vi "recenter.vi"() -> ()   [LabVIEW 2011]
doc: "This VI is an example of how to use the Host VI to open the I2C bus, write, read, and close I2C bus. This VI should work for any I2C EEPROM or RAM IC. Note that many of these devices have a limit on how many bytes can be writen to the device at a time.\n\nWritten By:\nPeter Fuller\nSenior Engineer\nplf Consulting, LLC\n\nemail: peter@plfconsulting.com\nphone: 617.699.2201"
uses:
  <vilib>/Platform/TimedLoop/XDataNode/timing_clust.ctl
  <vilib>/Platform/TimedLoop/XDataNode/nitl_modes.ctl
  <vilib>/Platform/TimedLoop/XDataNode/wakeup.ctl
  initialization/micron_globals.vi
  <vilib>/Platform/TimedLoop/XDataNode/XDataNode.xnode
  <vilib>/Platform/TimedLoop/XDataNode/XDNodeRunTimeDep.lvlib
panel:
  out "Waveform Chart":sgl[][](graph)
  out "Stalled axis":bool[](array[boolean])
  in  "Moved threshold":i16=20
  out "Error":sgl format="%#.0f"
  out "Running":bool
  out "Axis":i32
  in  "Max error":i16=100
  in  "Pulse count":i16=1000
  in  "Stop":bool
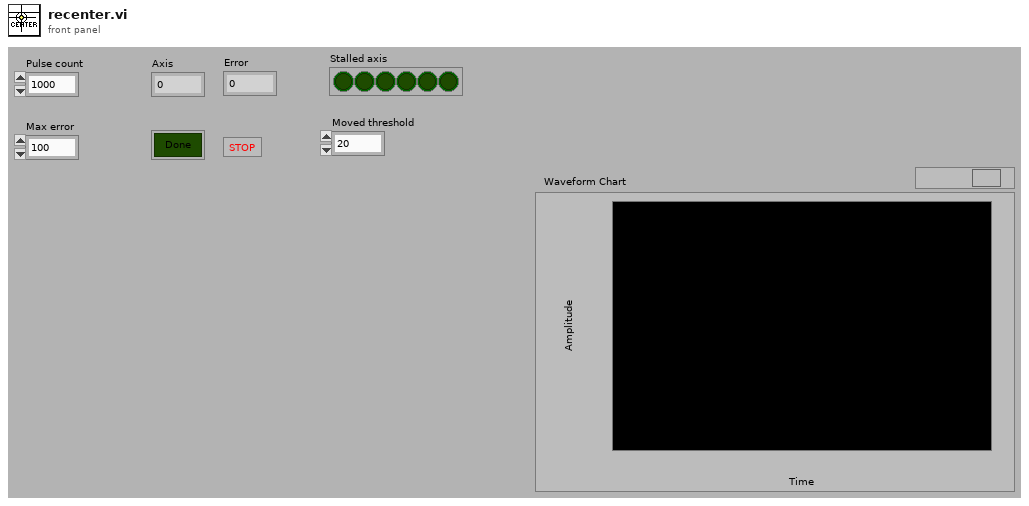
[diagram p1: front panel]
types:
  T1 = typedef "XDNodeRunTimeDep.lvlib/timing_clust.ctl" = cluster{"Expected End [f-1]":u64, "Actual End [f-1]":u64, "Finished Late? [f-1]":bool, "Expected End [i-1]":u64, "Actual End [i-1]":u64, "Finished Late? [i-1]":bool, "Expected Start [i]":u64, "Actual Start [i]":u64, "Expected Start [f]":u64, "Actual Start [f]":u64, "Source Name":string, "Structure Name":string, "Period":i64, "Deadline":i64, "Offset":i64, "Start":i64, "Priority":i32, "Timeout":i32, "Mode":T2, "Wakeup Reason":T3, "Error":errorcluster, "Source Type":string, "Secondary Source Type":string, "Global End Time":u64, "Global Start Time":u64, "Frame Duration":u64, "Iteration Duration":u64, "Assigned CPU":i32, "I/O Scan Engine Mode":u32}
  T2 = typedef "XDNodeRunTimeDep.lvlib/nitl_modes.ctl" = enum32{"No Change", "Process missed periods, maintain original phase", "Discard missed periods, maintain original phase", "Process missed periods, ignore original phase", "Discard missed periods, ignore original phase"}
  T3 = typedef "XDNodeRunTimeDep.lvlib/wakeup.ctl" = enum32{"Normal", "Aborted", "Asynchronous wakeup", "Timing source error", "Timed loop error", "Timeout"}
  T4 = typedef "Micron params.ctl" = cluster{"Stimulus":T5, "Goal Filter A":T7, "Mode controls":T8, "Manipulator type":enum16{"Current piezo", "Voltage piezo"}, "Manipulator calibration":T9, "Network":T11, "Goal Filter B":T7, "Cancellation":T12, "Transition time":sgl, "Estimation":T13}
  T5 = typedef "stimulus.ctl" = cluster{"Type":enum16{"Off", "Step", "Sine", "Triangle", "Arbitrary"}, "Phase":dbl, "Amplitude":sgl[], "Injection point":T6, "Closed loop":bool, "Offset":sgl[], "Tip -> world":bool, "Frequency":dbl, "Length":dbl}
  T6 = typedef "injection_point.ctl" = enum16{"Total pose", "V limiter", "Goal ", "Link position", "Link rate", "Link residue", "Link goal", "Link error", "Controller", "Output", "Drive", "DAC"}
  T7 = typedef "goal_loop_parms.ctl" = cluster{"Speedup max":sgl, "Speedup thresh":sgl, "Speedup nonlin":sgl, "Filters":cluster{"Lower Fc":sgl, "Lower Q":sgl, "Scale factor":sgl, "Upper Fc":sgl, "Upper Q":sgl, "V limit":sgl, "V limit range":sgl}[]}
  T8 = typedef "mode_conrols.ctl" = cluster{"Hold":bool, "Cancellation":bool, "Goal filter":bool, "Trigger":bool}
  T9 = typedef "manipulator_cal.ctl" = cluster{"Tool offsets":sgl[][], "Tip light calibration":T10, "Axial filter":cluster{"filter structure":enum32{"IIR 2nd Order", "IIR 4th Order"}, "Reverse Coefficients":dbl[], "Forward Coefficients":dbl[]}, "Lateral filter":cluster{"filter structure":enum32{"IIR 2nd Order", "IIR 4th Order"}, "Reverse Coefficients":dbl[], "Forward Coefficients":dbl[]}, "Handle light calibration":T10, "Base pivots":sgl[][], "Output pivots":sgl[][], "Length center":sgl, "Workspace height":sgl[], "Workspace diameter":sgl[], "Linearization":sgl[][], "Stack travel":sgl, "Saturation pos":sgl}
  T10 = typedef "probe_calibration.ctl" = sgl[][]
  T11 = typedef "network_params.ctl" = cluster{"Remote Host":string, "Send Status":bool, "Send Port":u16, "Recv Commands":bool, "Recv Port":u16}
  T12 = typedef "sq_control_params.ctl" = cluster{"KP":sgl, "KI":sgl, "KD":sgl, "Max vel":sgl, "Max acc":sgl, "Int error limit":dbl, "RCM gain":sgl, "Bypass":bool}
  T13 = typedef "estimation_controls.ctl" = cluster{"Link":cluster{"Measure noise":dbl[], "Process noise":dbl[], "Innovation limit":dbl[], "Enable":bool}, "Handle":cluster{"Measure noise":dbl[], "Process noise":dbl[], "State limits":dbl[], "Innovation limit":dbl[], "Prediction Lookahead":sgl, "Enable":bool}}
  T14 = typedef "micron_config.ctl" = cluster{"rt fifo":refnum<k33>, "Analog output task":refnum<k21>, "Analog output task 2":refnum<k21>, "Stimulus AO task":refnum<k21>, "Low-rate AIN task":refnum<k21>, "Pedal out task":refnum<k21>, "Pedal in task":refnum<k21>, "Loop timing source":string, "Relay out task":refnum<k21>, "Send UDP Conn":refnum<k16>, "Recv UDP Conn":refnum<k16>, "Host Addr":dbl, "I2C interface":T15, "trace_start notifier":refnum<notifier>, "trace_done notifier":refnum<notifier>, "ASAP FIFO":refnum<k33>}
  T15 = typedef "i2c_interface.ctl" = cluster{"FPGA VI Reference":T16}
  T16 = typedef "fpga_reference.ctl" = refnum<k20>
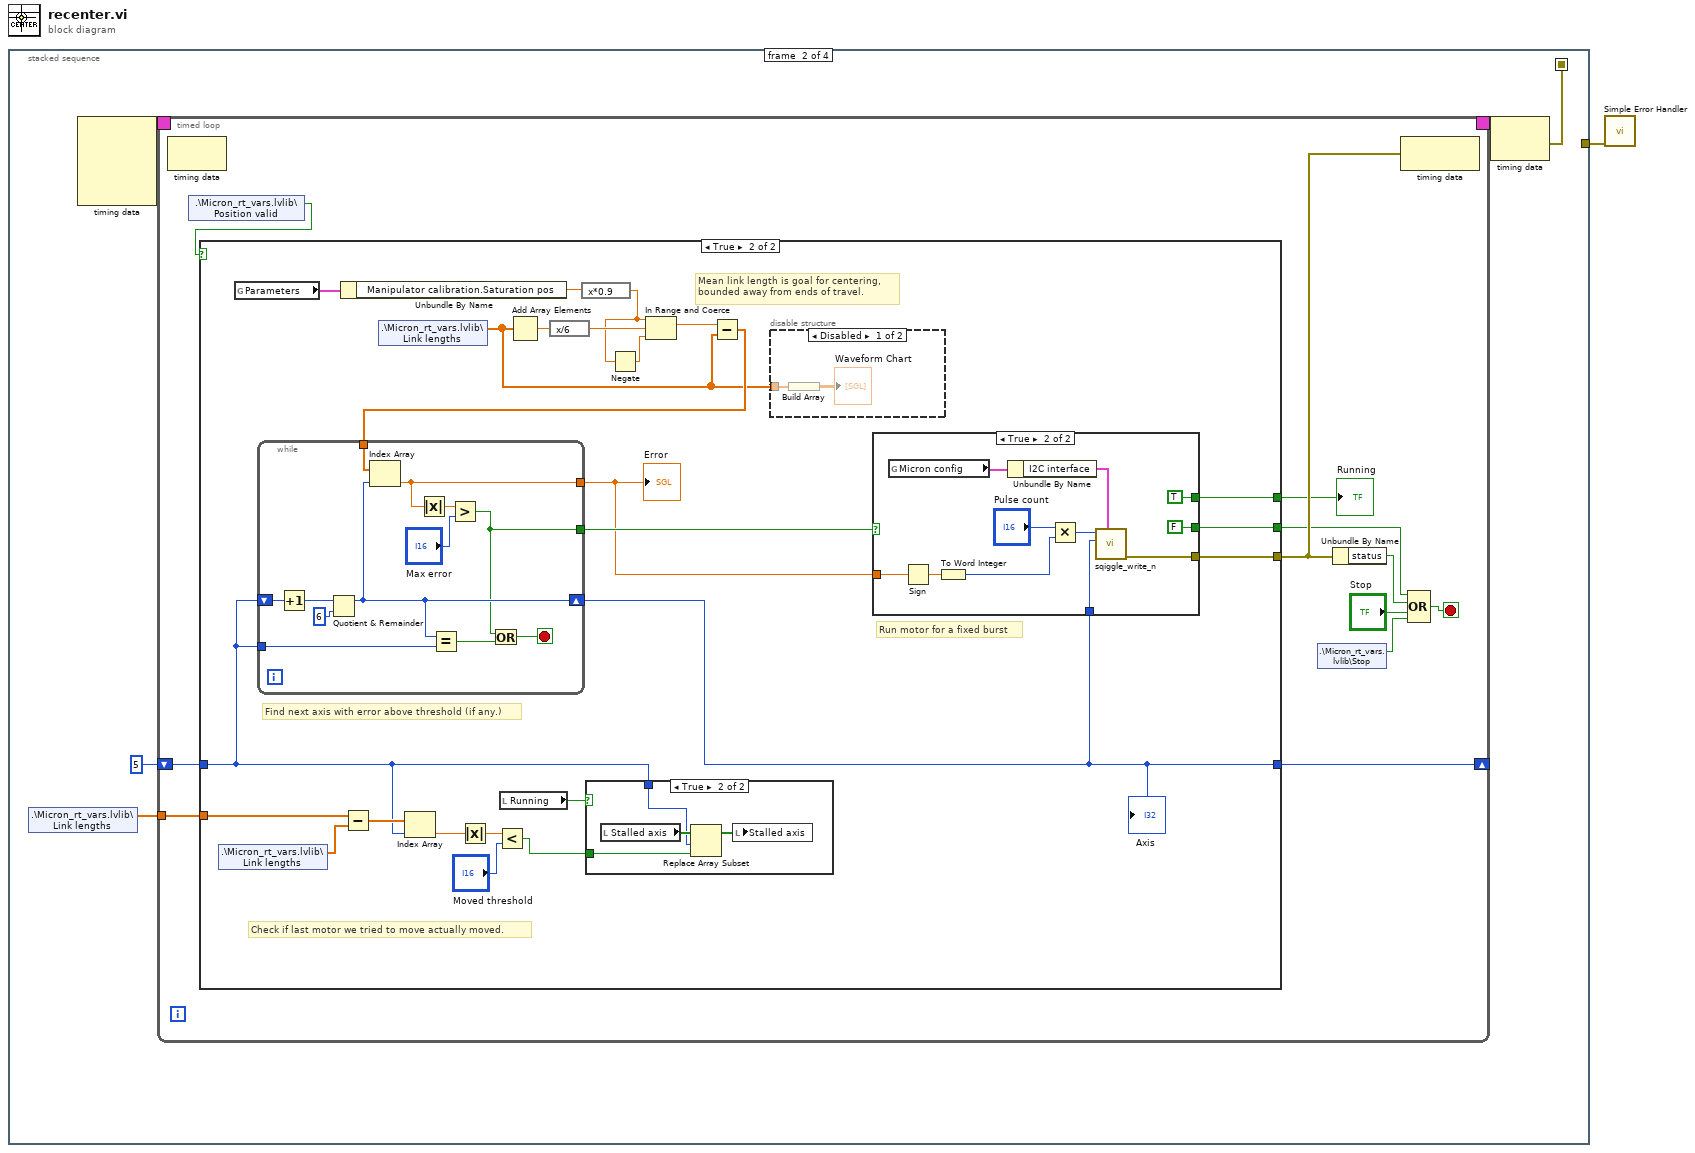
[diagram p0: block diagram]
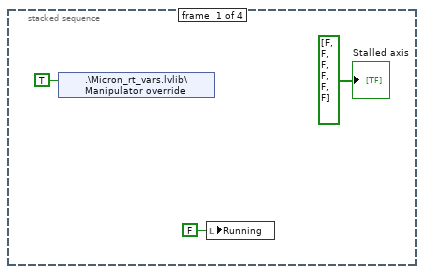
[diagram p2: hidden frame]
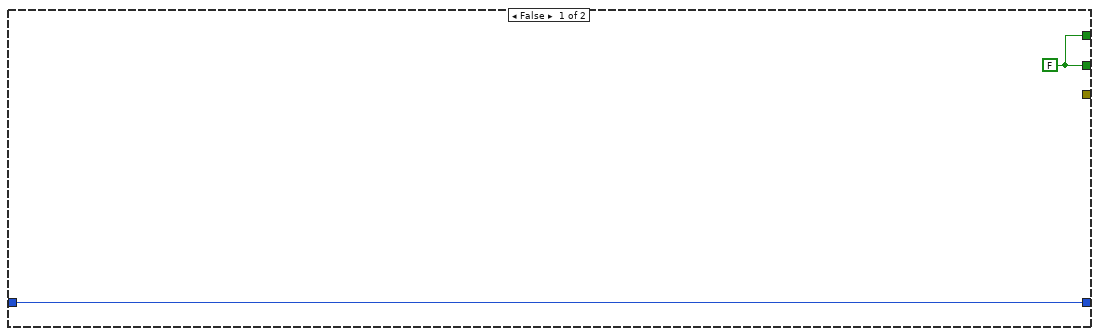
[diagram p3: hidden frame]
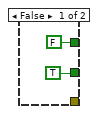
[diagram p6: hidden frame]
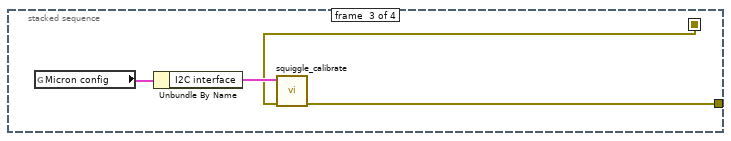
[diagram p7: hidden frame]
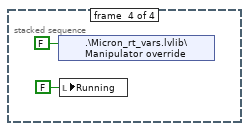
[diagram p8: hidden frame]
diagram:
  n1 = stacked-sequence {
    seq-local: [_ w7 _ _] -> [_ _ w86 _]
    tunnel: [_ _ w85 _] -> w1
    frame #0 {
      n2 = shared-variable ".\\Micron_rt_vars.lvlib\\Manipulator override"(TRUE ("Manipulator override")) -> ()  [unwired: 1 in, 1 out]
      n3 = local write "Running"(FALSE ("Running")) -> ()
      "Stalled axis" <- bool[] [FALSE, FALSE, FALSE, FALSE, FALSE, FALSE] ("Stalled axis")
    }
    frame #1 {
      n4 = shared-variable ".\\Micron_rt_vars.lvlib\\Link lengths"() -> (w6:sgl[])  [unwired: 1 in, 1 out]
      n5 = node-c288() -> (w9:T1)  [unwired: 4 in]
      n6 = timed-loop {
        timing: w9 -> [_]
        timing-out: [_] -> w8
        tunnel: w6 -> [w11]
        shift-right: [w12] -> _
        shift-left: 5 -> [w13]
        stop <- w19 stop-if-true
        n7 = node-c288() -> ()  [unwired: 1 in, 1 out]
        n8 = shared-variable ".\\Micron_rt_vars.lvlib\\Position valid"() -> (w10:bool)  [unwired: 1 in, 1 out]
        n9 = case shown="True" w10 {
          tunnel: [_ w46] -> w16
          tunnel: [w22 w38] -> w15
          tunnel: [w22 w37] -> w14
          tunnel: w13 -> [w21 w29]
          tunnel: [w21 w36] -> w12
          tunnel: w11 -> [_ w34]
          frame False {
            w22 = FALSE ("Running")
          }
          frame True {
            # "Check if last motor we tried to move actually moved."
            # "Run motor for a fixed burst"
            # "Find next axis with error above threshold (if any.)"
            # "Mean link length is goal for centering,\nbounded away from ends of travel."
            n10 = shared-variable ".\\Micron_rt_vars.lvlib\\Link lengths"() -> (w24:sgl[])  [unwired: 1 in, 1 out]
            n11 = global read "micron_globals.vi" "Parameters"() -> (w44:T4)
            n12 = Unbundle By Name(w44) -> ("Manipulator calibration.Saturation pos"=w43:sgl)
            n13 = Subtract(x=w34, y=w24) -> (x-y=w31:sgl[])
            n14 = shared-variable ".\\Micron_rt_vars.lvlib\\Link lengths"() -> (w23:sgl[])  [unwired: 1 in, 1 out]
            n15 = Index Array(array=w31, index=w29) -> (element=w30:sgl)
            n16 = Absolute Value(x=w30) -> (abs(x)=w33:sgl)
            n17 = Less?(x=w33, y="Moved threshold") -> (x < y?=w26:bool)
            n18 = local read "Running"() -> (w27:bool)
            n19 = Add Array Elements(numeric array=w23) -> (sum=w45:sgl)
            n20 = expression code="x/6"(w45) -> (w42:sgl)
            n21 = expression code="x*0.9"(w43) -> (w40:sgl)
            n22 = case shown="True" w27 {
              tunnel: w29 -> [_ w51]
              tunnel: w26 -> [_ w49]
              frame False {
              }
              frame True {
                n23 = local read "Stalled axis"() -> (w52:bool[])
                n24 = Replace Array Subset(array=w52, new element=w49, index=w51) -> (w50:bool[])
                n25 = local write "Stalled axis"(w50) -> ()
              }
            }
            n26 = Negate(x=w40) -> (-x=w41:sgl)
            n27 = In Range and Coerce(upper limit=w40, x=w42, lower limit=w41) -> (coerced(x)=w39:sgl)  [unwired: 1 out]
            n28 = Subtract(x=w39, y=w23) -> (x-y=w25:sgl[])
            n29 = while {
              shift-right: [w57] -> w36
              shift-left: w29 -> [w62]
              tunnel: w29 -> [w59]
              tunnel: w25 -> [w58]
              tunnel: [w54] -> w28
              tunnel: [w53] -> w35
              stop <- w55 stop-if-true
              n30 = Increment(x=w62) -> (x+1=w61:i32)
              n31 = Quotient & Remainder(x=w61, y=6) -> (x-y*floor(x/y)=w57:i32)  [unwired: 1 out]
              n32 = Index Array(array=w58, index=w57) -> (element=w54:sgl)
              n33 = Absolute Value(x=w54) -> (abs(x)=w63:sgl)
              n34 = Equal?(x=w57, y=w59) -> (x = y?=w56:bool)
              n35 = Greater?(x=w63, y="Max error") -> (0:w53:bool)
              n36 = Or(x=w53, y=w56) -> (x .or. y?=w55:bool)
            }
            "Axis" <- w36
            "Error" <- w28
            n37 = disable-structure shown="Disabled" {
              disable-tunnel: w23 -> [w47 _]
              frame Disabled {
                n38 = Build Array(w47) -> (→"Waveform Chart":sgl[][])
              }
              frame Enabled {
              }
            }
            n39 = case shown="True" w35 {
              tunnel: [_ w75] -> w46
              tunnel: w28 -> [_ w67]
              tunnel: w36 -> [_ w72]
              tunnel: [FALSE ("Running") TRUE ("Running")] -> w38
              tunnel: [TRUE ("Running") FALSE ("Running")] -> w37
              frame False {
              }
              frame True {
                n40 = global read "micron_globals.vi" "Micron config"() -> (w77:T14)
                n41 = Sign(1:w67) -> (0:w69:sgl)
                n42 = To Word Integer(number=w69) -> (16bit integer=w68:i16)
                n43 = Unbundle By Name(w77) -> ("I2C interface"=w76:T15)
                n44 = Multiply(x="Pulse count", y=w68) -> (x*y=w73:i16)
                n45 = call "sqiggle_write_n.vi"("I2C interface"=w76, "Axis num"=w72, "Pulse count"=w73) -> ("error out"=w75:errorcluster)  [unwired: 8 in]
              }
            }
          }
        }
        "Running" <- w15
        n46 = shared-variable ".\\Micron_rt_vars.lvlib\\Stop"() -> (w18:bool)  [unwired: 2 out]
        n47 = Unbundle By Name(w16) -> ("status"=w17:bool)
        n48 = node-c288(w16) -> ()  [unwired: 1 out]
        n49 = Compound Arithmetic op=OR(w14, w17, "Stop", w18) -> (w19:bool)
      }
      n50 = node-c288(w8) -> (w7:errorcluster)
    }
    frame #2 {
      n51 = global read "micron_globals.vi" "Micron config"() -> (w88:T14)
      n52 = Unbundle By Name(w88) -> ("I2C interface"=w87:T15)
      n53 = call "squiggle_calibrate.vi"("error in"=w86, "I2C interface"=w87) -> ("error out"=w85:errorcluster)  [unwired: 9 in]
    }
    frame #3 {
      n54 = shared-variable ".\\Micron_rt_vars.lvlib\\Manipulator override"(FALSE ("Manipulator override")) -> ()  [unwired: 1 in, 1 out]
      n55 = local write "Running"(FALSE ("Running")) -> ()
    }
  }
  n56 = call <vilib>:"Simple Error Handler.vi"("error in (no error)"=w1) -> ()  [unwired: 4 in, 5 out]
